vi "DataToStringArray.vi"(10 "MeasureMode":T1, 11 "MeasureData":T2) -> (3 "Array":string[](array[string]))   [LabVIEW 2012]
uses:
  Interface/MeasureModeControl.ctl
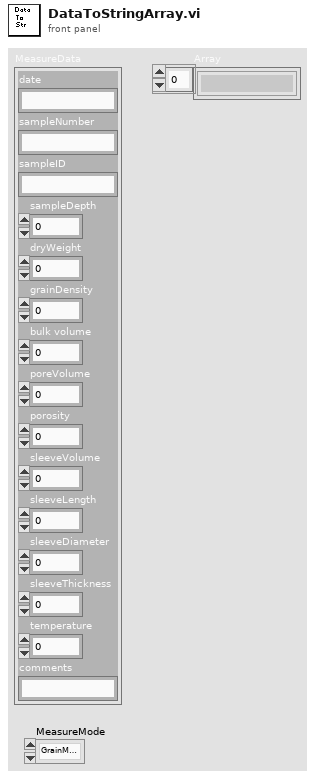
[diagram p1: front panel]
types:
  T1 = typedef "MeasureModeControl.ctl" = enum16{"GrainMeasure", "PoreMeasure"}
  T2 = cluster{"date":string, "sampleNumber":string, "sampleID":string, "sampleDepth":dbl, "dryWeight":dbl, "grainDensity":dbl, "bulk volume":dbl, "poreVolume":dbl, "porosity":dbl, "sleeveVolume":dbl, "sleeveLength":dbl, "sleeveDiameter":dbl, "sleeveThickness":dbl, "temperature":dbl, "comments":string}
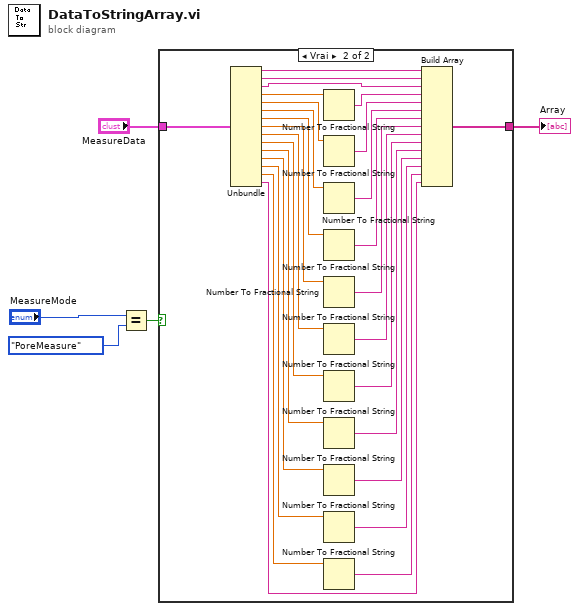
[diagram p0: block diagram]
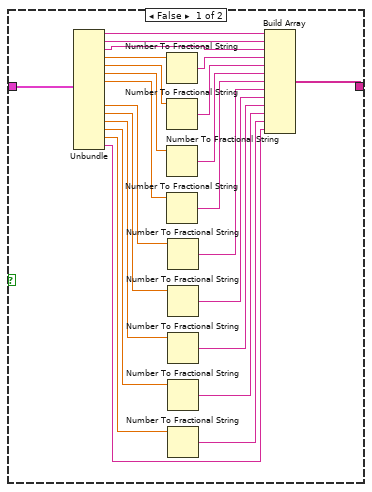
[diagram p2: hidden frame]
diagram:
  n1 = Equal?(x="MeasureMode", y=MeasureModeControl."PoreMeasure") -> (x = y?=w3:bool)
  n2 = case shown="Vrai" w3 {
    tunnel: [w12 w57] -> w5
    tunnel: "MeasureData" -> [w13 w50]
    frame False {
      n3 = Unbundle(w13) -> ("date"=w14:string, "sampleNumber"=w15:string, "sampleID"=w27:string, "sampleDepth"=w24:dbl, "dryWeight"=w25:dbl, "grainDensity"=w26:dbl, "bulk volume"=w22:dbl, "sleeveVolume"=w20:dbl, "sleeveLength"=w19:dbl, "sleeveDiameter"=w18:dbl, "sleeveThickness"=w16:dbl, "temperature"=w17:dbl, "comments"=w6:string)  [unwired: 2 out]
      n4 = Number To Fractional String(number=w24) -> (F-format string=w28:string)  [unwired: 3 in]
      n5 = Number To Fractional String(number=w25) -> (F-format string=w29:string)  [unwired: 3 in]
      n6 = Number To Fractional String(number=w26) -> (F-format string=w23:string)  [unwired: 3 in]
      n7 = Number To Fractional String(number=w22) -> (F-format string=w21:string)  [unwired: 3 in]
      n8 = Number To Fractional String(number=w20) -> (F-format string=w11:string)  [unwired: 3 in]
      n9 = Number To Fractional String(number=w19) -> (F-format string=w10:string)  [unwired: 3 in]
      n10 = Number To Fractional String(number=w18) -> (F-format string=w9:string)  [unwired: 3 in]
      n11 = Number To Fractional String(number=w16) -> (F-format string=w8:string)  [unwired: 3 in]
      n12 = Number To Fractional String(number=w17) -> (F-format string=w7:string)  [unwired: 3 in]
      n13 = Build Array(w14, w15, w27, w28, w29, w23, w21, w11, w10, w9, w8, w7, w6) -> (w12:string[])
    }
    frame True {
      n14 = Unbundle(w50) -> ("date"=w30:string, "sampleNumber"=w31:string, "sampleID"=w54:string, "sampleDepth"=w51:dbl, "dryWeight"=w52:dbl, "grainDensity"=w53:dbl, "bulk volume"=w48:dbl, "poreVolume"=w46:dbl, "porosity"=w45:dbl, "sleeveVolume"=w44:dbl, "sleeveLength"=w43:dbl, "sleeveDiameter"=w42:dbl, "sleeveThickness"=w40:dbl, "temperature"=w41:dbl, "comments"=w32:string)
      n15 = Number To Fractional String(number=w51) -> (F-format string=w55:string)  [unwired: 3 in]
      n16 = Number To Fractional String(number=w52) -> (F-format string=w56:string)  [unwired: 3 in]
      n17 = Number To Fractional String(number=w53) -> (F-format string=w49:string)  [unwired: 3 in]
      n18 = Number To Fractional String(number=w48) -> (F-format string=w47:string)  [unwired: 3 in]
      n19 = Number To Fractional String(number=w46) -> (F-format string=w39:string)  [unwired: 3 in]
      n20 = Number To Fractional String(number=w45) -> (F-format string=w38:string)  [unwired: 3 in]
      n21 = Number To Fractional String(number=w44) -> (F-format string=w37:string)  [unwired: 3 in]
      n22 = Number To Fractional String(number=w43) -> (F-format string=w36:string)  [unwired: 3 in]
      n23 = Number To Fractional String(number=w42) -> (F-format string=w35:string)  [unwired: 3 in]
      n24 = Number To Fractional String(number=w40) -> (F-format string=w34:string)  [unwired: 3 in]
      n25 = Number To Fractional String(number=w41) -> (F-format string=w33:string)  [unwired: 3 in]
      n26 = Build Array(w30, w31, w54, w55, w56, w49, w47, w39, w38, w37, w36, w35, w34, w33, w32) -> (w57:string[])
    }
  }
  "Array" <- w5
